vi "DSF.Engine.Memory.Buffer.Dispose.vi"(8 "error in (no error)":errorcluster, 11 "Buffer in":refnum<class "DSF.Engine.Memory.Buffer.lvclass">) -> (0 "error out":errorcluster)   [LabVIEW 2016, in "DSF.Engine.lvlib" / "DSF.Engine.Memory.Buffer.lvclass"]
uses:
  DSF.Engine.Memory.Buffer.lvclass
  C:/Git/SourceTree/DSF/Source/Submodules/Memory Manager/Source/Classes/Pointer.Internal/Memory.Pointer.Internal.lvclass
  Submodules/Memory Manager/Source/Classes/Pointer.Internal/Memory.Pointer.Internal.lvclass
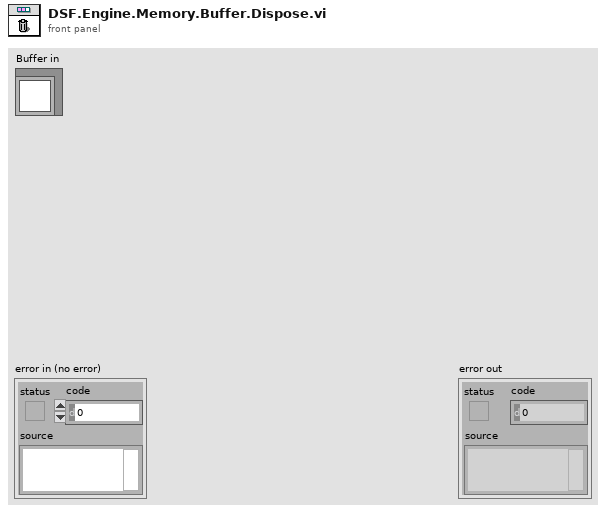
[diagram p1: front panel]
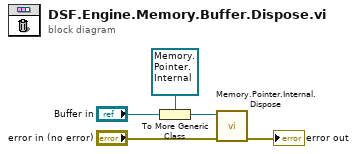
[diagram p0: block diagram]
diagram:
  n1 = To More Generic Class(target class=refnum<class "Memory.Pointer.Internal.lvclass"> refnum ("pointer"), reference="Buffer in") -> (generic class reference=w2:refnum<class "Memory.Pointer.Internal.lvclass">)
  n2 = call "Memory.Pointer.Internal.Dispose.vi"("error in (no error)"="error in (no error)", "pointer"=w2) -> ("error out"=→"error out":errorcluster)  [unwired: 9 in]
